vi "JSON elem to Complex.vi"(8 "error in (no error)":errorcluster, 11 "JSON in":string) -> (0 "error out":errorcluster, 3 "Numeric":cdb)   [LabVIEW 2018]
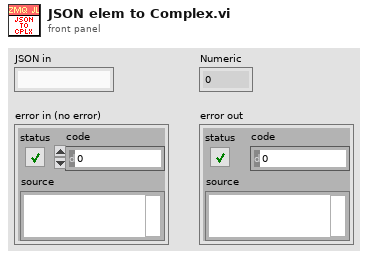
[diagram p1: front panel]
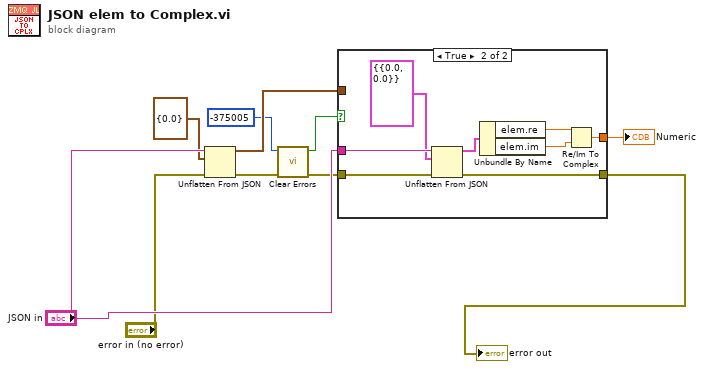
[diagram p0: block diagram]
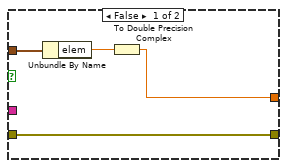
[diagram p2: hidden frame]
diagram:
  n1 = Unflatten From JSON(JSON string="JSON in", type and defaults=cluster{"elem":dbl} {"elem"=0.0} ("parsed response"), error in (no error)="error in (no error)") -> (value=w6:cluster{"elem":dbl}, error out=w2:errorcluster)  [unwired: 4 in]
  n2 = call <vilib>:"Clear Errors.vi"("error in (no error)"=w2, "specific error code to clear (0: all)"=-375005) -> ("error out"=w7:errorcluster, "specific error cleared?"=w5:bool)  [unwired: 4 in]
  n3 = case shown="True" w5 {
    tunnel: w7 -> [w14 w22]
    tunnel: w6 -> [w13 _]
    tunnel: "JSON in" -> [_ w20]
    tunnel: [w14 w21] -> w9
    tunnel: [w11 w15] -> w10
    frame False {
      n4 = Unbundle By Name(w13) -> ("elem"=w12:dbl)
      n5 = To Double Precision Complex(1:w12) -> (0:w11:cdb)
    }
    frame True {
      n6 = Unflatten From JSON(JSON string=w20, type and defaults=cluster{"elem":cluster{"re":dbl, "im":dbl}} {"elem"={"re"=0.0, "im"=0.0}}, error in (no error)=w22) -> (value=w18:cluster{"elem":cluster{"re":dbl, "im":dbl}}, error out=w21:errorcluster)  [unwired: 4 in]
      n7 = Unbundle By Name(w18) -> ("elem.re"=w17:dbl, "elem.im"=w16:dbl)
      n8 = Re/Im To Complex(1:w16, 2:w17) -> (0:w15:cdb)
    }
  }
  "Numeric" <- w10
  "error out" <- w9
